vi "Read_CMOD_SOFT_pkop250.vi"(8 "errin":errorcluster, 11 "CmodId":u32=1) -> (0 "error out":errorcluster caption="errout", 3 "SN":string)   [LabVIEW 2020]
uses:
  C/Program Files (x86)/National Instruments/LabVIEW 2020/user.lib/PCAN Basic/Controls/BaudrateEenum.ctl
  C/Program Files (x86)/National Instruments/LabVIEW 2020/user.lib/PCAN Basic/Controls/Channel.ctl
  C/Program Files (x86)/National Instruments/LabVIEW 2020/user.lib/PCAN Basic/PCANBasic.lvlib
panel:
  out "MDP OK":bool
  out "IDOK":bool
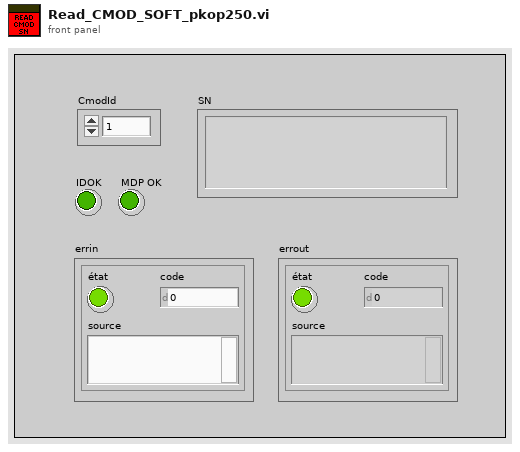
[diagram p1: front panel]
types:
  T1 = typedef "PCANBasic.lvlib/Channel.ctl" = enum16{"PCAN_NONEBUS", "not used1", "not used2", "not used3", "not used4", "not used5", "not used6", "not used7", "not used8", "not used9", "not used10", "not used11", "not used12", "not used13", "not used14", "not used15", "not used16", "not used17", "not used18", "not used19", "not used20", "not used21", "not used22", "not used23", "not used24", "not used25", "not used26", "not used27", "not used28", "not used29", "not used30", "not used31", "not used32", "PCAN_ISABUS1", "PCAN_ISABUS2", "PCAN_ISABUS3", "PCAN_ISABUS4", "PCAN_ISABUS5", "PCAN_ISABUS6", "PCAN_ISABUS7", "PCAN_ISABUS8", "not used41", "not used42", "not used43", "not used44", "not used45", "not used46", "not used47", "not used48", "PCAN_DNGBUS1", "not used50", "not used51", "not used52", "not used53", "not used54", "not used55", "not used56", "not used57", "not used58", "not used59", "not used60", "not used61", "not used62", "not used63", "not used64", "PCAN_PCIBUS1", "PCAN_PCIBUS2", "PCAN_PCIBUS3", "PCAN_PCIBUS4", "PCAN_PCIBUS5", "PCAN_PCIBUS6", "PCAN_PCIBUS7", "PCAN_PCIBUS8", "not used73", "not used74", "not used75", "not used76", "not used77", "not used78", "not used79", "not used80", "PCAN_USBBUS1", "PCAN_USBBUS2", "PCAN_USBBUS3", "PCAN_USBBUS4", "PCAN_USBBUS5", "PCAN_USBBUS6", "PCAN_USBBUS7", "PCAN_USBBUS8", "Not used89", "Not used90", "Not used91", "Not used92", "Not used93", "Not used94", "Not used95", "Not used96", "PCAN_PCCBUS1", "PCAN_PCCBUS2"}
  T2 = typedef "PCANBasic.lvlib/BaudrateEenum.ctl" = enum16{"CAN_Baud_1M", "CAN_Baud_800K", "CAN_BAUD_500K", "CAN_BAUD_250K", "CAN_BAUD_125K", "CAN_BAUD_100K", "CAN_BAUD_95K", "CAN_BAUD_83K", "CAN_BAUD_50K", "CAN_BAUD_47K", "CAN_BAUD_33K", "CAN_BAUD_20K", "CAN_BAUD_10K", "CAN_BAUD_5K", "User Baudrate"}
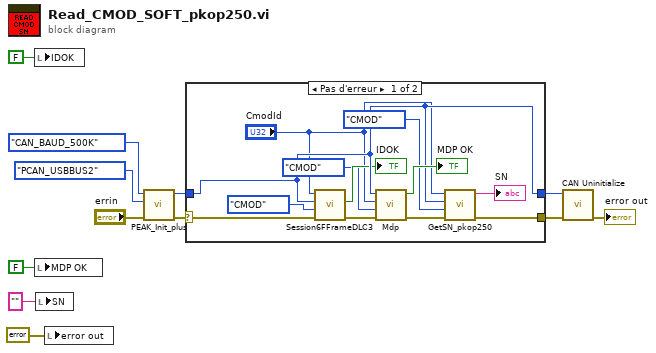
[diagram p0: block diagram]
diagram:
  n1 = local write "IDOK"(FALSE ("IDOK")) -> ()
  n2 = local write "MDP OK"(FALSE ("MDP OK")) -> ()
  n3 = local write "SN"("" ("SN")) -> ()
  n4 = local write "error out"(errorcluster {"status"=FALSE, "code"=0, "source"=""} ("error out")) -> ()
  n5 = call "PEAK_Init_plus.vi"("errin"="errin", "Channel"=Channel."PCAN_USBBUS2", "BTR0BTR1"=BaudrateEenum."CAN_BAUD_500K") -> ("errout"=w7:errorcluster, "Channel out"=w6:T1)  [unwired: 7 in]
  n6 = case shown="Pas d'erreur" w7 {
    selector: w7 -> [w19 w26]
    tunnel: [w22 w26] -> w11
    tunnel: w6 -> [w18 w25]
    tunnel: [w18 w25] -> w5
    frame No Error {
      n7 = call "Session6FFrameDLC3.vi"("errin"=w19, "Énum"=enum16{"PDU", "CMOD"}."CMOD", "ChanelIn"=w18, "IDnumber"="CmodId") -> ("errout"=w17:errorcluster, "Identique"=→"IDOK":bool)  [unwired: 4 in, 2 out]
      n8 = call "Mdp.vi"("errin"=w17, "Énum"=enum16{"PDU", "CMOD"}."CMOD", "CMODNum"="CmodId", "Channel out"=w18) -> ("errout"=w23:errorcluster, "OK"=→"MDP OK":bool)  [unwired: 6 in]
      n9 = call "GetSN_pkop250.vi"("err in"=w23, "TypeCible"=enum16{"CMOD", "BMS", "PDU"}."CMOD", "Channel in"=w18, "ECU Numb"="CmodId") -> ("errout"=w22:errorcluster, "Chaîne"=→"SN":string)  [unwired: 6 in]
    }
    frame Error {
    }
  }
  n10 = call "CAN Uninitialize.vi"("error in (no error)"=w11, "Channel"=w5) -> ("error out"=→"error out":errorcluster)  [unwired: 7 in, 2 out]
